vi "Go straight.vi"(10 "Distance Feet":dbl, 11 "RobotDriveDevRef in":T1) -> (3 "RobotDriveDevRef out":T1)   [LabVIEW 2017]
uses:
  <vilib>/Rock Robotics/WPI/RobotDrive/WPI_RobotDriveDevRef.ctl
  <vilib>/Rock Robotics/WPI/MotorControl/WPI_MotorControlDeviceRef.ctl
  <vilib>/Rock Robotics/WPI/MotorControl/WPI_MotorControlType.ctl
  <vilib>/Rock Robotics/SystemInterfaces/DIO/FPGA_DIOPWMChannel.ctl
  <vilib>/Rock Robotics/WPI/PWM/WPI_PWMDeadband.ctl
  <vilib>/Rock Robotics/SystemInterfaces/DIO/FPGA_DIOChannel.ctl
  <vilib>/Rock Robotics/WPI/SafetyOutput/WPI_SafetyOutputConfigMenu.ctl
  <vilib>/Rock Robotics/WPI/ThirdParty/Phoenix-LabVIEW/Motor Controller/Get/CTRE_Phoenix_MotorController_GetQuadratureData.vi
panel:
  out "Whie Loop Counts":i32
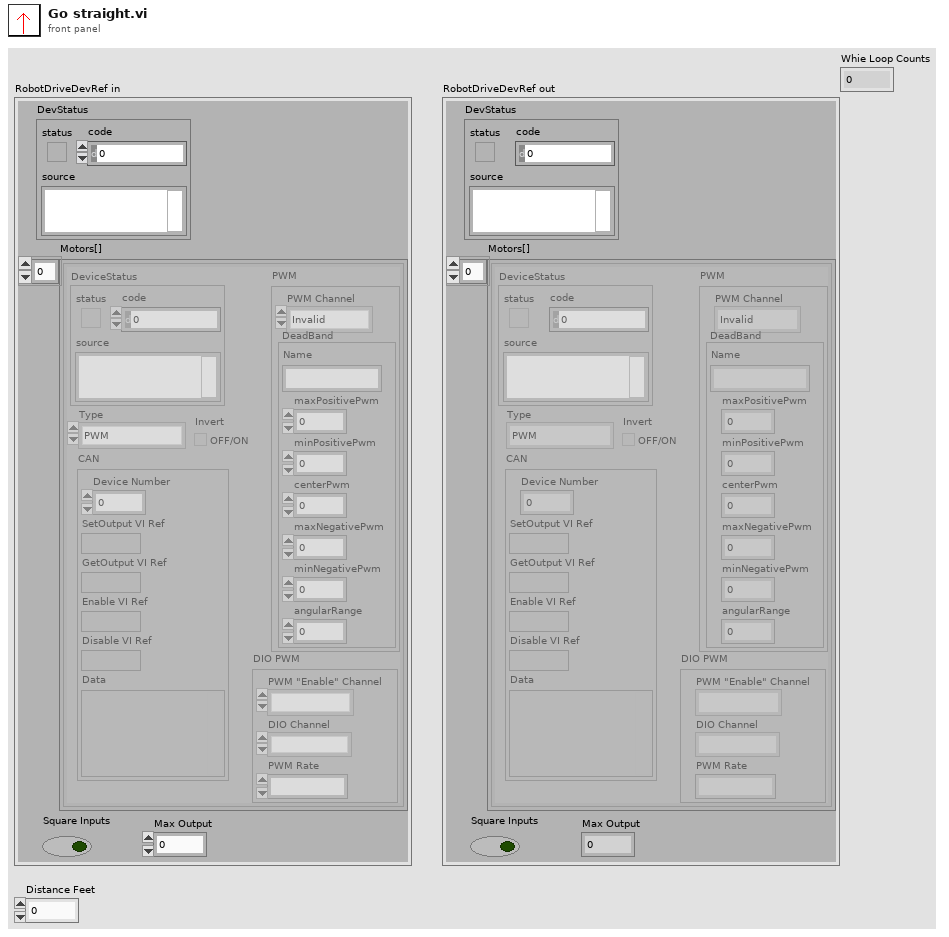
[diagram p1: front panel]
types:
  T1 = typedef "WPI_RobotDriveDevRef.ctl" = cluster{"DevStatus":errorcluster, "Motors[]":T2[], "Square Inputs":bool, "Max Output":dbl}
  T2 = typedef "WPI_MotorControlDeviceRef.ctl" = cluster{"DeviceStatus":errorcluster, "Type":T3, "PWM":cluster{"PWM Channel":T4, "DeadBand":T5}, "CAN":cluster{"Device Number":u8, "SetOutput VI Ref":variant, "GetOutput VI Ref":variant, "Enable VI Ref":variant, "Disable VI Ref":variant, "Data":variant}, "Invert":bool, "DIO PWM":cluster{"PWM \"Enable\" Channel":T4, "DIOChannel":T6, "PWM Rate":dbl}}
  T3 = typedef "WPI_MotorControlType.ctl" = enum16{"PWM", "CAN", "DIO PWM"}
  T4 = typedef "FPGA_DIOPWMChannel.ctl" = enum8{"PWM 0", "PWM 1", "PWM 2", "PWM 3", "PWM 4", "PWM 5", "PWM 6", "PWM 7", "PWM 8", "PWM 9", "PWM MXP 0", "PWM MXP 1", "PWM MXP 2", "PWM MXP 3", "PWM MXP 4", "PWM MXP 5", "PWM MXP 6", "PWM MXP 7", "PWM MXP 8", "PWM MXP 9", "Invalid"}
  T5 = typedef "WPI_PWMDeadband.ctl" = cluster{"Name":string, "maxPositivePwm":i32, "minPositivePwm":i32, "centerPwm":i32, "maxNegativePwm":i32, "minNegativePwm":i32, "angularRange":u16}
  T6 = typedef "FPGA_DIOChannel.ctl" = enum8{"DIO 0", "DIO 1", "DIO 2", "DIO 3", "DIO 4", "DIO 5", "DIO 6", "DIO 7", "DIO 8", "DIO 9", "DIO MXP 0", "DIO MXP 1", "DIO MXP 2", "DIO MXP 3", "DIO MXP 4", "DIO MXP 5", "DIO MXP 6", "DIO MXP 7", "DIO MXP 8", "DIO MXP 9", "DIO MXP 10", "DIO MXP 11", "DIO MXP 12", "DIO MXP 13", "DIO MXP 14", "DIO MXP 15", "SPI Port CS1", "SPI Port CS2", "SPI Port CS3", "SPI Port MISO", "SPI Port MOSI", "Invalid"}
  T7 = typedef "WPI_SafetyOutputConfigMenu.ctl" = enum16{"Enable", "Disable"}
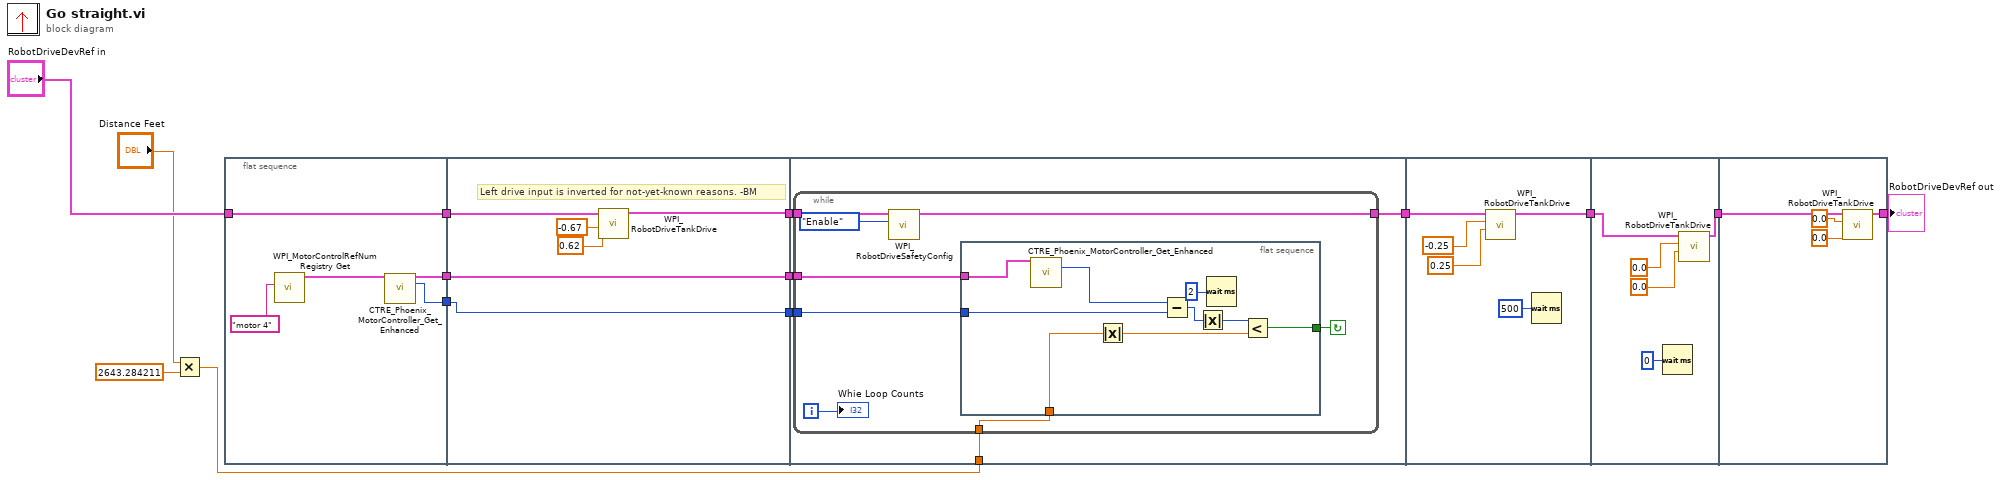
[diagram p0: block diagram]
diagram:
  n1 = Multiply(x="Distance Feet", y=2643.284211) -> (x*y=w5:dbl)
  n2 = flat-sequence {
    tunnel: "RobotDriveDevRef in" -> [w19]
    tunnel: [w19] -> w14
    tunnel: [w17] -> w13
    tunnel: [w15] -> w7
    tunnel: [w23] -> w12
    tunnel: [w25] -> w11
    tunnel: w14 -> [w24]
    tunnel: w13 -> [w25]
    tunnel: [w20] -> w8
    tunnel: w7 -> [w20]
    tunnel: [w28] -> w3
    tunnel: w12 -> [w30]
    tunnel: w11 -> [w29]
    tunnel: w8 -> [w27]
    tunnel: w5 -> [w26]
    tunnel: w3 -> [w49]
    tunnel: [w50] -> w2
    tunnel: w2 -> [w54]
    tunnel: [w53] -> w1
    tunnel: [w58] -> w9
    tunnel: w1 -> [w59]
    frame #0 {
      n3 = call <vilib>:"WPI_MotorControlRefNum Registry Get.vi"("refnum name"="motor 4") -> ("MotorControlDevRef"=w18:T2)  [unwired: 9 in, 1 out]
      n4 = call-poly <vilib>:"CTRE_Phoenix_MotorController_Get_Enhanced.vi"("PhoenixMotorControlDevRef"=w18) -> ("PhoenixMotorControlDevRef"=w17:T2, "Quadrature Position"=w15:i32)  [unwired: 11 in, 2 out]
    }
    frame #1 {
      # "Left drive input is inverted for not-yet-known reasons. -BM"
      n5 = call <vilib>:"WPI_RobotDriveTankDrive.vi"("Right axis value"=0.62, "Left axis value"=-0.67, "RobotDriveDevRef"=w24) -> ("RobotDriveDevRef"=w23:T1)  [unwired: 6 in, 2 out]
    }
    frame #2 {
      n6 = while {
        tunnel: w30 -> [w38]
        tunnel: w29 -> [w37]
        tunnel: [w35] -> w28
        tunnel: w27 -> [w33]
        tunnel: w26 -> [w32]
        i -> [w31]
        stop <- w36 continue-if-true
        n7 = call <vilib>:"WPI_RobotDriveSafetyConfig.vi"("mode"=WPI_SafetyOutputConfigMenu."Enable", "RobotDriveDevRef"=w38) -> ("RobotDriveDevRef"=w35:T1)  [unwired: 8 in, 1 out]
        n8 = flat-sequence {
          tunnel: w37 -> [w43]
          tunnel: [w46] -> w36
          tunnel: w33 -> [w45]
          tunnel: w32 -> [w41]
          frame #0 {
            n9 = call-poly <vilib>:"CTRE_Phoenix_MotorController_Get_Enhanced.vi"("PhoenixMotorControlDevRef"=w43) -> ("Quadrature Position"=w44:i32)  [unwired: 11 in, 3 out]
            n10 = Absolute Value(x=w41) -> (abs(x)=w42:dbl)
            n11 = Subtract(x=w44, y=w45) -> (x-y=w40:i32)
            n12 = Absolute Value(x=w40) -> (abs(x)=w39:i32)
            n13 = Wait (ms)(milliseconds to wait=u32 2) -> ()  [unwired: 1 out]
            n14 = Less?(x=w39, y=w42) -> (x < y?=w46:bool)
          }
        }
        "Whie Loop Counts" <- w31
      }
    }
    frame #3 {
      n15 = call <vilib>:"WPI_RobotDriveTankDrive.vi"("Right axis value"=0.25, "Left axis value"=-0.25, "RobotDriveDevRef"=w49) -> ("RobotDriveDevRef"=w50:T1)  [unwired: 6 in, 2 out]
      n16 = Wait (ms)(milliseconds to wait=u32 500) -> ()  [unwired: 1 out]
    }
    frame #4 {
      n17 = Wait (ms)(milliseconds to wait=u32 0) -> ()  [unwired: 1 out]
      n18 = call <vilib>:"WPI_RobotDriveTankDrive.vi"("Right axis value"=0.0, "Left axis value"=0.0, "RobotDriveDevRef"=w54) -> ("RobotDriveDevRef"=w53:T1)  [unwired: 6 in, 2 out]
    }
    frame #5 {
      n19 = call <vilib>:"WPI_RobotDriveTankDrive.vi"("Right axis value"=0.0, "Left axis value"=0.0, "RobotDriveDevRef"=w59) -> ("RobotDriveDevRef"=w58:T1)  [unwired: 6 in, 2 out]
    }
  }
  "RobotDriveDevRef out" <- w9
